vi "Benchmark_ExtractClusterElements.vi"() -> ()   [LabVIEW 2020]
uses:
  _built_ppls/OpenVariant.lvlibp
panel:
  out "Array":string[](array[string])
  out "Elements":variant[](array[variant])
  out "Waveform Chart":dbl(graph)
  out "execution time per call":dbl
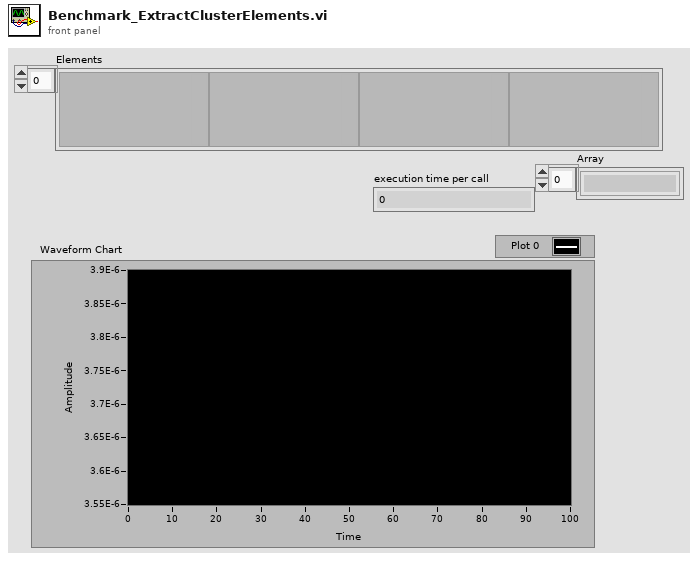
[diagram p1: front panel]
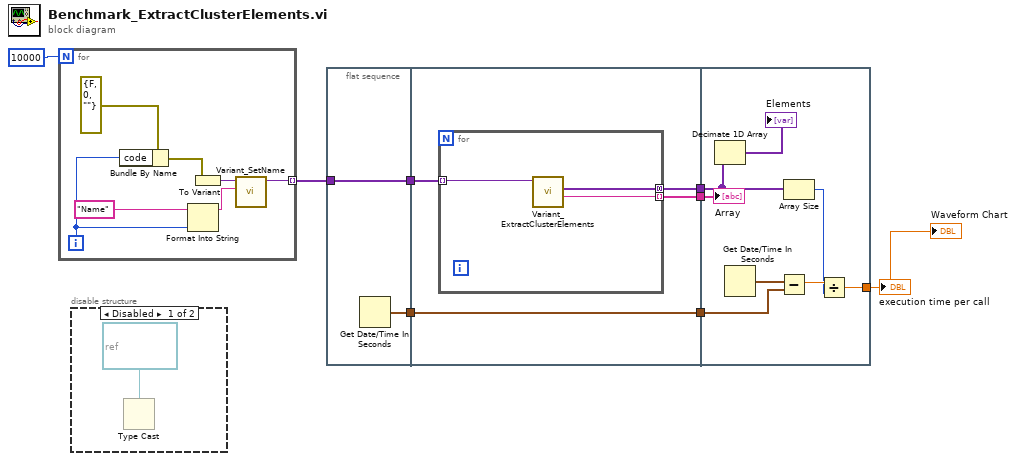
[diagram p0: block diagram]
diagram:
  n1 = for {
    N: 10000 -> [_]
    tunnel: [w12] -> w7 mode=indexing
    i -> [w10]
    n2 = Bundle By Name(cluster=errorcluster {"status"=FALSE, "code"=0, "source"=""} ("error constant"), "code"=w10) -> (w9:errorcluster)
    n3 = Format Into String(initial string="Name", w10) -> (resulting string=w13:string)  [unwired: 2 in, 1 out]
    n4 = To Variant(anything=w9) -> (Variant=w14:variant)
    n5 = call "Variant_SetName.vi"("Name"=w13, "Variant"=w14) -> ("Named Variant"=w12:variant)  [unwired: 9 in]
  }
  n6 = disable-structure shown="Disabled" {
    frame Disabled {
      n7 = Type Cast(type=refnum<queue> refnum ("queue out")) -> ()  [unwired: 1 in, 1 out]
    }
    frame Enabled {
    }
  }
  n8 = flat-sequence {
    tunnel: w7 -> [w18]
    tunnel: [w18] -> w6
    tunnel: [w17] -> w4
    tunnel: w6 -> [w22]
    tunnel: [w21] -> w5
    tunnel: w4 -> [w21]
    tunnel: [w20] -> w2
    tunnel: [w19] -> w1
    tunnel: w5 -> [w32]
    tunnel: [w29] -> w3
    tunnel: w2 -> [w27]
    tunnel: w1 -> [w26]
    frame #0 {
      n9 = Get Date/Time In Seconds() -> (seconds since 1Jan1904=w17:timestamp)
    }
    frame #1 {
      n10 = for {
        tunnel: w22 -> [w25] mode=indexing
        tunnel: [w24] -> w20 mode=concatenating
        tunnel: [w23] -> w19 mode=indexing
        n11 = call "Variant_ExtractClusterElements.vi"("Cluster"=w25) -> ("name"=w23:string, "Elements"=w24:variant[])  [unwired: 8 in, 1 out]
      }
    }
    frame #2 {
      n12 = Decimate 1D Array(w27) -> (→"Elements":variant[])  [unwired: 2 out]
      n13 = Get Date/Time In Seconds() -> (seconds since 1Jan1904=w33:timestamp)
      n14 = Subtract(x=w33, y=w32) -> (x-y=w31:dbl)
      n15 = Array Size(array=w27) -> (size(s)=w30:i32)
      n16 = Divide(x=w31, y=w30) -> (x/y=w29:dbl)
      "Array" <- w26
    }
  }
  "execution time per call" <- w3
  "Waveform Chart" <- w3
